vi "Arm_Begin.vi"   [LabVIEW 2020]
uses:
  <vilib>/Rock Robotics/SystemInterfaces/DIO/FPGA_DIOChannel.ctl
  <vilib>/Rock Robotics/WPI/ThirdParty/REV Robotics/REVLib/Typedef/Spark MAX Absolute Encoder Average Depth Size.ctl
  Robot Global Data.vi
  <vilib>/Rock Robotics/WPI/Switch/WPI_SwitchOpenLimit.vi
types:
  T1 = typedef "Spark MAX Absolute Encoder Average Depth Size.ctl" = enum16{"1", "2", "4", "8", "16", "32", "64", "128"}
  T2 = typedef "FPGA_DIOChannel.ctl" = enum8{"DIO 0", "DIO 1", "DIO 2", "DIO 3", "DIO 4", "DIO 5", "DIO 6", "DIO 7", "DIO 8", "DIO 9", "DIO MXP 0", "DIO MXP 1", "DIO MXP 2", "DIO MXP 3", "DIO MXP 4", "DIO MXP 5", "DIO MXP 6", "DIO MXP 7", "DIO MXP 8", "DIO MXP 9", "DIO MXP 10", "DIO MXP 11", "DIO MXP 12", "DIO MXP 13", "DIO MXP 14", "DIO MXP 15", "SPI Port CS1", "SPI Port CS2", "SPI Port CS3", "SPI Port MISO", "SPI Port MOSI", "Invalid"}
  T3 = typedef "WPI_MotorControlDeviceRef.ctl" = cluster{"DeviceStatus":errorcluster, "Type":T4, "PWM":cluster{"PWM Channel":T5, "DeadBand":T6}, "CAN":cluster{"Device Number":u8, "SetOutput VI Ref":variant, "GetOutput VI Ref":variant, "Enable VI Ref":variant, "Disable VI Ref":variant, "Data":variant}, "Invert":bool, "DIO PWM":cluster{"PWM \"Enable\" Channel":T5, "DIOChannel":T2, "PWM Rate":dbl}}
  T4 = typedef "WPI_MotorControlType.ctl" = enum16{"PWM", "CAN", "DIO PWM"}
  T5 = typedef "FPGA_DIOPWMChannel.ctl" = enum8{"PWM 0", "PWM 1", "PWM 2", "PWM 3", "PWM 4", "PWM 5", "PWM 6", "PWM 7", "PWM 8", "PWM 9", "PWM MXP 0", "PWM MXP 1", "PWM MXP 2", "PWM MXP 3", "PWM MXP 4", "PWM MXP 5", "PWM MXP 6", "PWM MXP 7", "PWM MXP 8", "PWM MXP 9", "Invalid"}
  T6 = typedef "WPI_PWMDeadband.ctl" = cluster{"Name":string, "maxPositivePwm":i32, "minPositivePwm":i32, "centerPwm":i32, "maxNegativePwm":i32, "minNegativePwm":i32, "angularRange":u16}
  T7 = typedef "WPI_SwitchDevRef.ctl" = cluster{"DevStatus":errorcluster, "DIO Channel":T2, "CntIndex":T8, "Normally Closed":bool}
  T8 = typedef "FPGA_CounterCtrSystemIndex.ctl" = enum8{"Ctr 0", "Ctr 1", "Ctr 2", "Ctr 3", "Ctr 4", "Ctr 5", "Ctr 6", "Ctr 7", "Invalid"}
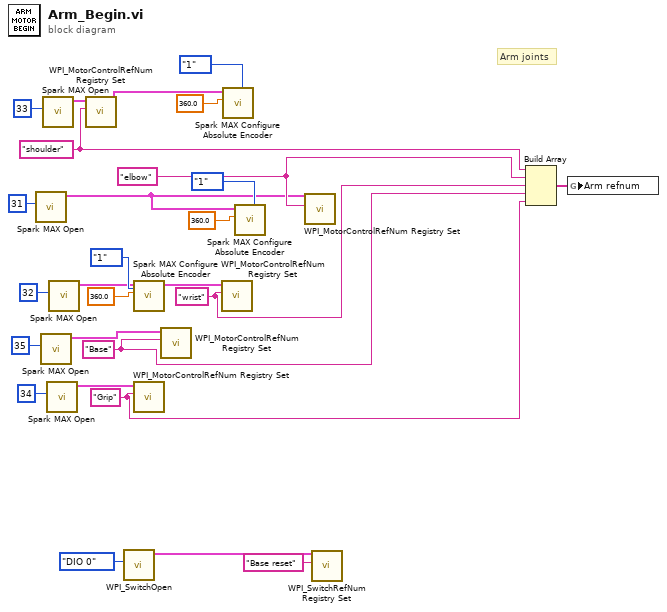
[diagram p0: block diagram]
diagram:
  w4 = "Grip" ("refnum name")
  w5 = "Base" ("refnum name")
  w15 = "wrist" ("refnum name")
  w14 = "elbow" ("refnum name")
  w26 = "shoulder" ("refnum name")
  # "Arm joints"
  n1 = call <vilib>:"Spark MAX Open.vi"("Device Number"=u8 31) -> ("MotorControlDeviceRef"=w1:T3)  [unwired: 9 in, 1 out]
  n2 = call <vilib>:"Spark MAX Open.vi"("Device Number"=u8 35) -> ("MotorControlDeviceRef"=w21:T3)  [unwired: 9 in, 1 out]
  n3 = call <vilib>:"Spark MAX Open.vi"("Device Number"=u8 33) -> ("MotorControlDeviceRef"=w22:T3)  [unwired: 9 in, 1 out]
  n4 = call <vilib>:"Spark MAX Open.vi"("Device Number"=u8 34) -> ("MotorControlDeviceRef"=w12:T3)  [unwired: 9 in, 1 out]
  n5 = call <vilib>:"Spark MAX Open.vi"("Device Number"=u8 32) -> ("MotorControlDeviceRef"=w17:T3)  [unwired: 9 in, 1 out]
  n6 = call <vilib>:"WPI_MotorControlRefNum Registry Set.vi"("refnum name"=w26, "MotorControlDevRef"=w22) -> ("MotorControlDevRef"=w9:T3)  [unwired: 8 in, 1 out]
  n7 = call-poly <vilib>:"WPI_SwitchOpen.vi"("DIO Channel"=FPGA_DIOChannel."DIO 0") -> ("SwitchDevRef"=w8:T7)  [unwired: 9 in, 1 out]
  n8 = call <vilib>:"Spark MAX Configure Absolute Encoder.vi"("Average Depth (128)"=Spark_MAX_Absolute_Encoder_Average_Depth_Size."1", "Position Conversion Factor (1)"=360.0, "MotorControlDeviceRef in"=w17) -> ("MotorControlDeviceRef out"=w16:T3)  [unwired: 7 in, 1 out]
  n9 = call <vilib>:"WPI_MotorControlRefNum Registry Set.vi"("refnum name"=w4, "MotorControlDevRef"=w12) -> ()  [unwired: 8 in, 2 out]
  n10 = call <vilib>:"WPI_MotorControlRefNum Registry Set.vi"("refnum name"=w5, "MotorControlDevRef"=w21) -> ()  [unwired: 8 in, 2 out]
  n11 = call <vilib>:"WPI_MotorControlRefNum Registry Set.vi"("refnum name"=w15, "MotorControlDevRef"=w16) -> ()  [unwired: 8 in, 2 out]
  n12 = call <vilib>:"Spark MAX Configure Absolute Encoder.vi"("Average Depth (128)"=Spark_MAX_Absolute_Encoder_Average_Depth_Size."1", "Position Conversion Factor (1)"=360.0, "MotorControlDeviceRef in"=w9) -> ()  [unwired: 7 in, 2 out]
  n13 = call <vilib>:"Spark MAX Configure Absolute Encoder.vi"("Average Depth (128)"=Spark_MAX_Absolute_Encoder_Average_Depth_Size."1", "Position Conversion Factor (1)"=360.0, "MotorControlDeviceRef in"=w1) -> ()  [unwired: 7 in, 2 out]
  n14 = call <vilib>:"WPI_MotorControlRefNum Registry Set.vi"("refnum name"=w14, "MotorControlDevRef"=w1) -> ()  [unwired: 8 in, 2 out]
  n15 = call <vilib>:"WPI_SwitchRefNum Registry Set.vi"("refnum name"="Base reset", "SwitchDevRef"=w8) -> ()  [unwired: 8 in, 2 out]
  n16 = Build Array(w26, w14, w15, w5, w4) -> (w27:string[])
  n17 = global write "Robot Global Data.vi" "Arm refnum"(w27) -> ()
